vi "Read Multi Eval Meas Trace ES Flatness Results.vi"(8 "error in (no error)":errorcluster, 10 "Instance (1)":T1=1, 11 "VISA resource name":refnum<visa-resource-name>) -> (0 "error out":errorcluster, 1 "Trace ES Flatness Results":dbl[](array[numeric]) format="%^.3e", 2 "Reliability":i32, 3 "VISA resource name out":refnum<visa-resource-name>)   [LabVIEW 2020, in "Rohde&Schwarz CMXP NR FR2 Measurement.lvlib"]
doc: "Starts a new single shot measurement and returns the multi eval measurement trace ES Flatness results.\n\nAttribute:\nRSCMXPNRFR2M_ATTR_READ_MULTI_EVAL_MEASUREMENT_TRACE_ESF_RESULTS\n\nRemote-control command:\nREAD:NRMMw:MEAS<i>:MEValuation:TRACe:ESFLatness?"
uses:
  <instrlib>/Rohde&Schwarz CMXP NR FR2 Measurement/Rohde&Schwarz CMXP NR FR2 Measurement.lvlib
  <instrlib>/Rohde&Schwarz CMXP NR FR2 Measurement/Private/_Instance.ctl
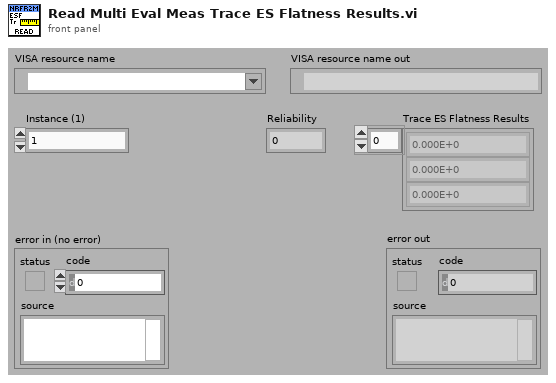
[diagram p1: front panel]
types:
  T1 = typedef "Rohde&Schwarz CMXP NR FR2 Measurement.lvlib/_Instance.ctl" = i32
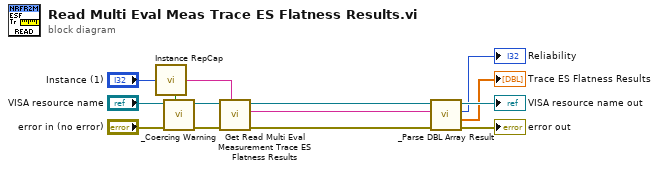
[diagram p0: block diagram]
diagram:
  n1 = call <instrlib>:"Instance RepCap.vi"("Instance In"="Instance (1)") -> ("In Range?"=w3:bool, "RepCap Identifier Out"=w8:string)  [unwired: 1 in]
  n2 = call <instrlib>:"_Coercing Warning.vi"("In Range?"=w3, "error in (no error)"="error in (no error)", "VISA resource name"="VISA resource name") -> ("error out"=w4:errorcluster, "VISA resource name out"=w5:refnum<visa-resource-name>)  [unwired: 7 in]
  n3 = call "Get Read Multi Eval Measurement Trace ES Flatness Results"("Repeated Capabilities"=w8, "error in (no error)"=w4, "instrument handle"=w5) -> ("error out"=w14:errorcluster, "Read Multi Eval Measurement Trace ES Flatness Results"=w10:string, "instrument handle out"=w13:refnum<visa-resource-name>)  [unwired: 6 in]
  n4 = call <instrlib>:"_Parse DBL Array Result.vi"("error in (no error)"=w14, "Input String"=w10, "VISA resource name"=w13) -> ("error out"=→"error out":errorcluster, "Results"=→"Trace ES Flatness Results":dbl[], "Reliability"=→"Reliability":i32, "VISA resource name out"=→"VISA resource name out":refnum<visa-resource-name>)  [unwired: 5 in]
